vi "Simulate Error.vi"(8 "error in (no error)":errorcluster, 11 "Actor Tests in":refnum<class "Actor Tests.lvclass">) -> (0 "error out":errorcluster, 3 "Actor Tests out":refnum<class "Actor Tests.lvclass">)   [LabVIEW 2020, in "Actor Tests.lvlib" / "Actor Tests.lvclass"]
uses:
  Actor Tests.lvclass
  Actor Tests.lvclass/Actor Tests.ctl
  <vilib>/ErrorRing/Error Ring.xnode
  <vilib>/Utility/error.llb/Error Cluster From Error Code.vi
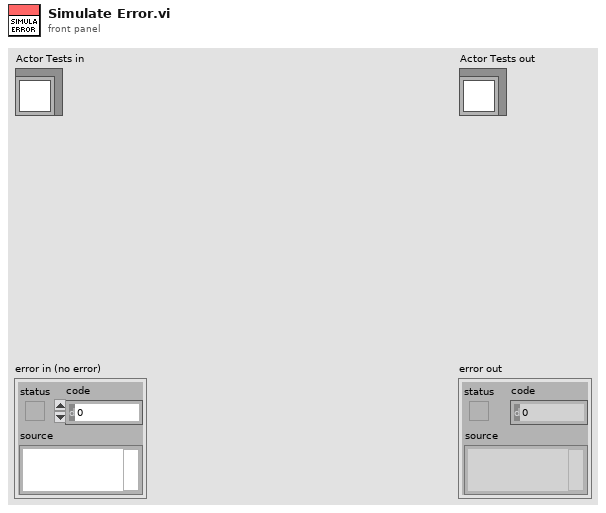
[diagram p1: front panel]
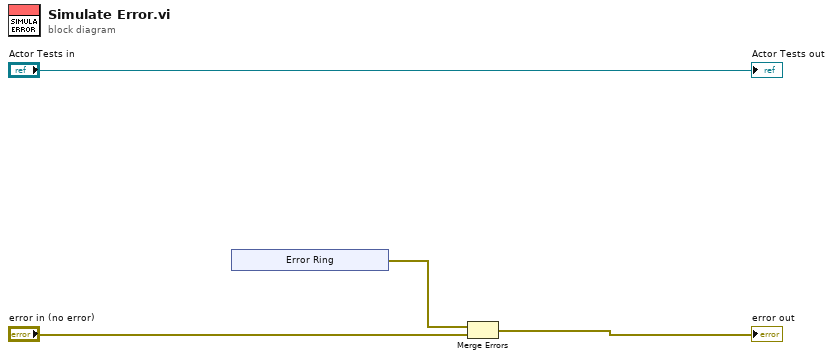
[diagram p0: block diagram]
diagram:
  n1 = xnode "Error Ring"() -> ("error out"=w1:errorcluster)
  n2 = Merge Errors(w1, "error in (no error)") -> (→"error out":errorcluster)
  "Actor Tests out" <- "Actor Tests in"
